vi "Func-엑셀 데이터를 그래프로 출력.vi"() -> ()   [LabVIEW 2015] (continued)
-18.3\t-18.31\t-8.468\n-18.3\t-18.31\t-8.468\n-18.3\t-18.31\t-8.468\n-18.3\t-18.31\t-8.469\n-18.3\t-18.31\t-8.468\n-18.3\t-18.31\t-8.47\n-18.3\t-18.31\t-8.471\n-18.3\t-18.31\t-8.473\n-18.3\t-18.31\t-8.477\n-18.3\t-18.31\t-8.479\n-18.3\t-18.31\t-8.48\n-18.3\t-18.31\t-8.477\n-18.3\t-18.31\t-8.477\n-18.3\t-18.31\t-8.478\n-18.3\t-18.31\t-8.474\n-18.3\t-18.31\t-8.47\n-18.3\t-18.31\t-8.47\n-18.3\t-18.31\t-8.472\n-18.3\t-18.31\t-8.475\n-18.3\t-18.31\t-8.474\n-18.3\t-18.31\t-8.478\n-18.3\t-18.31\t-8.48\n-18.3\t-18.31\t-8.48\n-18.3\t-18.31\t-8.482\n-18.3\t-18.31\t-8.481\n-18.3\t-18.31\t-8.48\n-18.3\t-18.31\t-8.48\n-18.3\t-18.31\t-8.477\n-18.3\t-18.31\t-8.48\n-18.3\t-18.31\t-8.48\n-18.3\t-18.31\t-8.483\n-18.3\t-18.31\t-8.484\n-18.3\t-18.31\t-8.484\n-18.3\t-18.31\t-8.489\n-18.3\t-18.31\t-8.49\n-18.3\t-18.31\t-8.49\n-18.3\t-18.31\t-8.489\n-18.3\t-18.31\t-8.487\n-18.3\t-18.31\t-8.486\n-18.3\t-18.31\t-8.484\n-18.3\t-18.31\t-8.481\n-18.3\t-18.31\t-8.482\n-18.3\t-18.31\t-8.484\n-18.3\t-18.31\t-8.483\n-18.3\t-18.31\t-8.486\n-18.3\t-18.31\t-8.487\n-18.3\t-18.31\t-8.489\n-18.3\t-18.31\t-8.488\n-18.3\t-18.31\t-8.484\n-18.3\t-18.31\t-8.486\n-18.3\t-18.31\t-8.487\n-18.3\t-18.31\t-8.491\n-18.3\t-18.31\t-8.491\n-18.3\t-18.31\t-8.491\n-18.3\t-18.31\t-8.495\n-18.3\t-18.31\t-8.496\n-18.3\t-18.31\t-8.492\n-18.3\t-18.31\t-8.491\n-18.3\t-18.31\t-8.493\n-18.3\t-18.31\t-8.496\n-18.3\t-18.31\t-8.495\n-18.3\t-18.31\t-8.495\n-18.3\t-18.31\t-8.496\n-18.3\t-18.31\t-8.495\n-18.3\t-18.31\t-8.497\n-18.3\t-18.31\t-8.494\n-18.3\t-18.31\t-8.495\n-18.3\t-18.31\t-8.5\n-18.3\t-18.31\t-8.499\n-18.3\t-18.31\t-8.5\n-18.3\t-18.31\t-8.499\n-18.3\t-18.31\t-8.503\n-18.3\t-18.31\t-8.507\n-18.3\t-18.31\t-8.505\n-18.3\t-18.31\t-8.507\n-18.3\t-18.31\t-8.506\n-18.3\t-18.31\t-8.506\n-18.3\t-18.31\t-8.503\n-18.3\t-18.31\t-8.502\n-18.3\t-18.31\t-8.503\n-18.3\t-18.31\t-8.503\n-18.3\t-18.31\t-8.505\n-18.3\t-18.31\t-8.504\n-18.3\t-18.31\t-8.507\n-18.3\t-18.31\t-8.502\n-18.3\t-18.31\t-8.5\n-18.3\t-18.31\t-8.502\n-18.3\t-18.31\t-8.505\n-18.3\t-18.31\t-8.508\n-18.3\t-18.31\t-8.506\n-18.3\t-18.31\t-8.508\n-18.3\t-18.31\t-8.511\n-18.3\t-18.31\t-8.514\n-18.3\t-18.31\t-8.513\n-18.3\t-18.31\t-8.512\n-18.3\t-18.31\t-8.515\n-18.3\t-18.31\t-8.517\n-18.3\t-18.31\t-8.513\n-18.3\t-18.31\t-8.509\n-18.3\t-18.31\t-8.508\n-18.3\t-18.31\t-8.509\n-18.3\t-18.31\t-8.507\n-18.3\t-18.31\t-8.507\n-18.393\t-18.38\t-8.775\n-18.477\t-18.44\t-8.782\n-18.56\t-18.33\t-8.786\n-18.643\t-18.35\t-8.786\n-18.727\t-18.4\t-8.796\n-18.81\t-18.46\t-8.785\n-18.893\t-18.53\t-8.79\n-18.977\t-18.6\t-8.793\n-19.06\t-18.68\t-8.792\n-19.143\t-18.77\t-8.794\n-19.227\t-18.87\t-8.797\n-19.31\t-18.99\t-8.789\n-19.393\t-19.09\t-8.798\n-19.477\t-19.21\t-8.807\n-19.56\t-19.33\t-8.797\n-19.643\t-19.43\t-8.805\n-19.727\t-19.53\t-8.807\n-19.81\t-19.65\t-8.809\n-19.893\t-19.77\t-8.82\n-19.977\t-19.88\t-8.813\n-20.06\t-20.01\t-8.825\n-20.143\t-20.12\t-8.83\n-20.227\t-20.24\t-8.835\n-20.31\t-20.34\t-8.841\n-20.393\t-20.46\t-8.852\n-20.477\t-20.57\t-8.857\n-20.56\t-20.68\t-8.861\n-20.643\t-20.8\t-8.873\n-20.727\t-20.9\t-8.873\n-20.81\t-21.01\t-8.89\n-20.893\t-21.11\t-8.904\n-20.977\t-21.21\t-8.911\n-21.06\t-21.33\t-8.929\n-21.143\t-21.43\t-8.927\n-21.227\t-21.54\t-8.944\n-21.31\t-21.63\t-8.961\n-21.393\t-21.71\t-8.978\n-21.477\t-21.8\t-8.993\n-21.56\t-21.87\t-9.011\n-21.643\t-21.94\t-9.028\n-21.727\t-22.01\t-9.045\n-21.81\t-22.07\t-9.071\n-21.893\t-22.14\t-9.091\n-21.977\t-22.21\t-9.109\n-22.06\t-22.28\t-9.134\n-22.143\t-22.36\t-9.152\n-22.227\t-22.45\t-9.172\n-22.31\t-22.53\t-9.2\n-22.393\t-22.6\t-9.224\n-22.477\t-22.68\t-9.25\n-22.56\t-22.76\t-9.272\n-22.643\t-22.84\t-9.297\n-22.727\t-22.92\t-9.329\n-22.81\t-22.99\t-9.355\n-22.893\t-23.07\t-9.387\n-22.977\t-23.15\t-9.423\n-23.06\t-23.22\t-9.445\n-23.143\t-23.29\t-9.477\n-23.227\t-23.36\t-9.505\n-23.31\t-23.45\t-9.534\n-23.393\t-23.53\t-9.572\n-23.477\t-23.62\t-9.603\n-23.56\t-23.69\t-9.63\n-23.643\t-23.77\t-9.668\n-23.727\t-23.85\t-9.7\n-23.81\t-23.93\t-9.739\n-23.893\t-24.01\t-9.771\n-23.977\t-24.09\t-9.805\n-24.06\t-24.17\t-9.846\n-24.143\t-24.24\t-9.882\n-24.227\t-24.31\t-9.915\n-24.31\t-24.4\t-9.965\n-24.393\t-24.49\t-10.003\n-24.477\t-24.56\t-10.039\n-24.56\t-24.64\t-10.073\n-24.643\t-24.72\t-10.12\n-24.727\t-24.81\t-10.156\n-24.81\t-24.88\t-10.202\n-24.893\t-24.96\t-10.24\n-24.977\t-25.04\t-10.284\n-25.06\t-25.1\t-10.323\n-25.143\t-25.19\t-10.372\n-25.227\t-25.27\t-10.418\n-25.31\t-25.35\t-10.457\n-25.393\t-25.42\t-10.498\n-25.477\t-25.5\t-10.549\n-25.56\t-25.58\t-10.6\n-25.643\t-25.65\t-10.641\n-25.727\t-25.74\t-10.692\n-25.81\t-25.83\t-10.733\n-25.893\t-25.91\t-10.783\n-25.977\t-26\t-10.832\n-26.06\t-26.08\t-10.873\n-26.143\t-26.15\t-10.932\n-26.227\t-26.24\t-10.976\n-26.31\t-26.32\t-11.023\n-26.393\t-26.41\t-11.073\n-26.477\t-26.48\t-11.118\n-26.56\t-26.56\t-11.17\n-26.643\t-26.65\t-11.228\n-26.727\t-26.73\t-11.275\n-26.81\t-26.81\t-11.33\n-26.893\t-26.88\t-11.382\n-26.977\t-26.96\t-11.434\n-27.06\t-27.05\t-11.488\n-27.143\t-27.13\t-11.539\n-27.227\t-27.21\t-11.586\n-27.31\t-27.29\t-11.647\n-27.393\t-27.37\t-11.699\n-27.477\t-27.45\t-11.745\n-27.56\t-27.52\t-11.804\n-27.643\t-27.62\t-11.864\n-27.727\t-27.7\t-11.916\n-27.81\t-27.79\t-11.971\n-27.893\t-27.87\t-12.027\n-27.977\t-27.95\t-12.079\n-28.06\t-28.03\t-12.136\n-28.143\t-28.11\t-12.201\n-28.227\t-28.2\t-12.257\n-28.31\t-28.27\t-12.312\n-28.393\t-28.34\t-12.365\n-28.477\t-28.41\t-12.42\n-28.56\t-28.49\t-12.481\n-28.643\t-28.57\t-12.543\n-28.727\t-28.62\t-12.597\n-28.81\t-28.69\t-12.665\n-28.893\t-28.77\t-12.714\n-28.977\t-28.84\t-12.777\n-29.06\t-28.94\t-12.842\n-29.143\t-29.01\t-12.898\n-29.227\t-29.09\t-12.951\n-29.31\t-29.16\t-13.021\n-29.393\t-29.23\t-13.081\n-29.477\t-29.3\t-13.142\n-29.56\t-29.38\t-13.202\n-29.643\t-29.47\t-13.272\n-29.727\t-29.54\t-13.326\n-29.81\t-29.61\t-13.389\n-29.893\t-29.69\t-13.455\n-29.977\t-29.75\t-13.518\n-30.06\t-29.82\t-13.585\n-30.143\t-29.89\t-13.646\n-30.227\t-29.97\t-13.701\n-30.31\t-30.04\t-13.77\n-30.393\t-30.11\t-13.834\n-30.477\t-30.17\t-13.901\n-30.56\t-30.25\t-13.957\n-30.643\t-30.33\t-14.017\n-30.727\t-30.41\t-14.083\n-30.81\t-30.47\t-14.148\n-30.893\t-30.53\t-14.214\n-30.977\t-30.61\t-14.278\n-31.06\t-30.69\t-14.342\n-31.143\t-30.77\t-14.413\n-31.227\t-30.85\t-14.474\n-31.31\t-30.93\t-14.534\n-31.393\t-30.99\t-14.599\n-31.477\t-31.07\t-14.666\n-31.56\t-31.14\t-14.736\n-31.643\t-31.2\t-14.794\n-31.727\t-31.28\t-14.858\n-31.81\t-31.34\t-14.926\n-31.893\t-31.4\t-14.989\n-31.977\t-31.47\t-15.061\n-32.06\t-31.54\t-15.121\n-32.143\t-31.59\t-15.184\n-32.227\t-31.65\t-15.247\n-32.31\t-31.72\t-15.306\n-32.393\t-31.78\t-15.383\n-32.477\t-31.84\t-15.443\n-32.56\t-31.91\t-15.514\n-32.643\t-31.98\t-15.58\n-32.727\t-32.04\t-15.645\n-32.81\t-32.12\t-15.707\n-32.893\t-32.19\t-15.763\n-32.977\t-32.26\t-15.84\n-33.06\t-32.32\t-15.909\n-33.143\t-32.38\t-15.976\n-33.227\t-32.45\t-16.038\n-33.31\t-32.5\t-16.112\n-33.393\t-32.57\t-16.169\n-33.477\t-32.63\t-16.237\n-33.56\t-32.71\t-16.298\n-33.643\t-32.77\t-16.368\n-33.727\t-32.83\t-16.44\n-33.81\t-32.89\t-16.507\n-33.893\t-32.95\t-16.564\n-33.977\t-33.01\t-16.636\n-34.06\t-33.07\t-16.703\n-34.143\t-33.13\t-16.773\n-34.227\t-33.18\t-16.849\n-34.31\t-33.24\t-16.907\n-34.393\t-33.3\t-16.971\n-34.477\t-33.35\t-17.047\n-34.56\t-33.42\t-17.107\n-34.643\t-33.48\t-17.175\n-34.727\t-33.55\t-17.237\n-34.81\t-33.6\t-17.304\n-34.893\t-33.65\t-17.37\n-34.977\t-33.71\t-17.43\n-35.06\t-33.77\t-17.502\n-35.143\t-33.81\t-17.574\n-35.227\t-33.87\t-17.633\n-35.31\t-33.93\t-17.701\n-35.393\t-33.99\t-17.767\n-35.477\t-34.04\t-17.843\n-35.56\t-34.1\t-17.901\n-35.643\t-34.17\t-17.968\n-35.727\t-34.23\t-18.035\n-35.81\t-34.28\t-18.101\n-35.893\t-34.33\t-18.162\n-35.977\t-34.39\t-18.234\n-36.06\t-34.45\t-18.304\n-36.143\t-34.51\t-18.366\n-36.227\t-34.57\t-18.426\n-36.31\t-34.62\t-18.493\n-36.393\t-34.69\t-18.558\n-36.477\t-34.74\t-18.622\n-36.56\t-34.79\t-18.701\n-36.643\t-34.84\t-18.761\n-36.727\t-34.9\t-18.83\n-36.81\t-34.96\t-18.904\n-36.893\t-35.02\t-18.953\n-36.977\t-35.07\t-19.021\n-37.06\t-35.12\t-19.084\n-37.143\t-35.17\t-19.152\n-37.227\t-35.22\t-19.221\n-37.31\t-35.28\t-19.285\n-37.393\t-35.33\t-19.348\n-37.477\t-35.38\t-19.409\n-37.56\t-35.44\t-19.473\n-37.643\t-35.5\t-19.538\n-37.727\t-35.56\t-19.6\n-37.81\t-35.61\t-19.672\n-37.893\t-35.67\t-19.735\n-37.977\t-35.73\t-19.793\n-38.06\t-35.77\t-19.856\n-38.143\t-35.83\t-19.925\n-38.227\t-35.87\t-19.992\n-38.31\t-35.91\t-20.059\n-38.393\t-35.97\t-20.12\n-38.477\t-36.03\t-20.18\n-38.56\t-36.08\t-20.245\n-38.643\t-36.13\t-20.312\n-38.727\t-36.18\t-20.375\n-38.81\t-36.22\t-20.427\n-38.893\t-36.29\t-20.506\n-38.977\t-36.33\t-20.566\n-39.06\t-36.38\t-20.625\n-39.143\t-36.44\t-20.691\n-39.227\t-36.5\t-20.754\n-39.31\t-36.55\t-20.818\n-39.393\t-36.6\t-20.882\n-39.477\t-36.65\t-20.931\n-39.56\t-36.71\t-21.005\n-39.643\t-36.77\t-21.066\n-39.727\t-36.82\t-21.126\n-39.81\t-36.88\t-21.179\n-39.893\t-36.93\t-21.246\n-39.977\t-36.98\t-21.304\n-40.06\t-37.04\t-21.37\n-40\t-37.1\t-21.425\n-40\t-37.1\t-21.426\n-40\t-37.11\t-21.432\n-40\t-37.11\t-21.436\n-40\t-37.11\t-21.443\n-40\t-37.12\t-21.441\n-40\t-37.13\t-21.448\n-40\t-37.13\t-21.453\n-40\t-37.14\t-21.456\n-40\t-37.15\t-21.467\n-40\t-37.16\t-21.473\n-40\t-37.16\t-21.486\n-40\t-37.17\t-21.496\n-40\t-37.17\t-21.499\n-40\t-37.17\t-21.505\n-40\t-37.18\t-21.511\n-40\t-37.18\t-21.516\n-40\t-37.18\t-21.52\n-40\t-37.18\t-21.521\n-40\t-37.19\t-21.527\n-40\t-37.19\t-21.534\n-40\t-37.19\t-21.543\n-40\t-37.2\t-21.549\n-40\t-37.2\t-21.555\n-40\t-37.2\t-21.564\n-40\t-37.21\t-21.571\n-40\t-37.21\t-21.573\n-40\t-37.22\t-21.578\n-40\t-37.22\t-21.583\n-40\t-37.23\t-21.59\n-40\t-37.23\t-21.598\n-40\t-37.24\t-21.605\n-40\t-37.24\t-21.613\n-40\t-37.25\t-21.616\n-40\t-37.25\t-21.618\n-40\t-37.25\t-21.623\n-40\t-37.26\t-21.628\n-40\t-37.26\t-21.631\n-40\t-37.26\t-21.638\n-40\t-37.26\t-21.648\n-40\t-37.27\t-21.655\n-40\t-37.27\t-21.664\n-40\t-37.28\t-21.672\n-40\t-37.28\t-21.679\n-40\t-37.29\t-21.686\n-40\t-37.3\t-21.687\n-40\t-37.3\t-21.695\n-40\t-37.31\t-21.696\n-40\t-37.32\t-21.7\n-40\t-37.32\t-21.707\n-40\t-37.33\t-21.715\n-40\t-37.33\t-21.725\n-40\t-37.33\t-21.73\n-40\t-37.33\t-21.741\n-40\t-37.34\t-21.746\n-40\t-37.34\t-21.753\n-40\t-37.35\t-21.759\n-40\t-37.36\t-21.764\n-40\t-37.36\t-21.772\n-40\t-37.37\t-21.777\n-40\t-37.37\t-21.781\n-40\t-37.38\t-21.785\n-40\t-37.38\t-21.795\n-40\t-37.39\t-21.802\n-40\t-37.4\t-21.805\n-40\t-37.4\t-21.816\n-40\t-37.41\t-21.821\n-40\t-37.41\t-21.824\n-40\t-37.41\t-21.829\n-40\t-37.41\t-21.831\n-40\t-37.42\t-21.837\n-40\t-37.42\t-21.843\n-40\t-37.43\t-21.849\n-40\t-37.43\t-21.859\n-40\t-37.44\t-21.869\n-40\t-37.44\t-21.879\n-40\t-37.45\t-21.883\n-40\t-37.45\t-21.892\n-40\t-37.46\t-21.896\n-40\t-37.47\t-21.898\n-40\t-37.47\t-21.902\n-40\t-37.48\t-21.901\n-40\t-37.48\t-21.904\n-40\t-37.48\t-21.909\n-40\t-37.49\t-21.916\n-40\t-37.49\t-21.921\n-40\t-37.49\t-21.927\n-40\t-37.49\t-21.937\n-40\t-37.5\t-21.947\n-40\t-37.51\t-21.956\n-40\t-37.52\t-21.961\n-40\t-37.53\t-21.966\n-40\t-37.54\t-21.977\n-40\t-37.54\t-21.978\n-40\t-37.55\t-21.98\n-40\t-37.56\t-21.986\n-40\t-37.56\t-21.989\n-40\t-37.57\t-21.995\n-40\t-37.57\t-22.001\n-40\t-37.58\t-22.008\n-40\t-37.59\t-22.015\n-40\t-37.59\t-22.022\n-40\t-37.6\t-22.027\n-40\t-37.61\t-22.035\n-40\t-37.61\t-22.039\n-40\t-37.62\t-22.048\n-40\t-37.63\t-22.052\n-40\t-37.63\t-22.061\n-40\t-37.63\t-22.066\n-40\t-37.64\t-22.071\n-40\t-37.64\t-22.076\n-40\t-37.64\t-22.079\n-40\t-37.64\t-22.086\n-40\t-37.65\t-22.088\n-40\t-37.65\t-22.096\n-40\t-37.66\t-22.105\n-40\t-37.66\t-22.111\n-40\t-37.67\t-22.118\n-40\t-37.67\t-22.125\n-40\t-37.68\t-22.132\n-40\t-37.68\t-22.138\n-40\t-37.69\t-22.145\n-40\t-37.69\t-22.154\n-40\t-37.7\t-22.157\n-40\t-37.71\t-22.165\n-40\t-37.71\t-22.168\n-40\t-37.71\t-22.17\n-40\t-37.71\t-22.177\n-40\t-37.71\t-22.18\n-40\t-37.72\t-22.186\n-40\t-37.72\t-22.192\n-40\t-37.73\t-22.198\n-40\t-37.74\t-22.203\n-40\t-37.75\t-22.207\n-40\t-37.75\t-22.213\n-40\t-37.76\t-22.219\n-40\t-37.77\t-22.227\n-40\t-37.77\t-22.233\n-40\t-37.78\t-22.241\n-40\t-37.78\t-22.251\n-40\t-37.79\t-22.256\n-40\t-37.79\t-22.263\n-40\t-37.79\t-22.271\n-40\t-37.79\t-22.276\n-40\t-37.8\t-22.279\n-40\t-37.8\t-22.286\n-40\t-37.81\t-22.289\n-40\t-37.82\t-22.294\n-40\t-37.82\t-22.298\n-40\t-37.83\t-22.306\n-40\t-37.83\t-22.31\n-40\t-37.84\t-22.318\n-40\t-37.84\t-22.325\n-40\t-37.85\t-22.33\n-40\t-37.86\t-22.341\n-40\t-37.86\t-22.342\n-40\t-37.86\t-22.346\n-40\t-37.87\t-22.352\n-40\t-37.87\t-22.358\n-40\t-37.88\t-22.362\n-40\t-37.88\t-22.369\n-40\t-37.88\t-22.377\n-40\t-37.89\t-22.386\n-40\t-37.9\t-22.393\n-40\t-37.91\t-22.398\n-40\t-37.91\t-22.403\n-40\t-37.92\t-22.408\n-40\t-37.92\t-22.413\n-40\t-37.93\t-22.42\n-40\t-37.93\t-22.43\n-40\t-37.93\t-22.432\n-40\t-37.94\t-22.441\n-40\t-37.94\t-22.447\n-40\t-37.94\t-22.453\n-40\t-37.95\t-22.454\n-40\t-37.95\t-22.458\n-40\t-37.96\t-22.466\n-40\t-37.97\t-22.47\n-40\t-37.97\t-22.476\n-40\t-37.98\t-22.482\n-40\t-37.98\t-22.492\n-40\t-37.99\t-22.496\n-40\t-37.99\t-22.5\n-40\t-38\t-22.505\n-40\t-38.01\t-22.511\n-40\t-38.01\t-22.515\n-40\t-38.01\t-22.521\n-40\t-38.02\t-22.527\n-40\t-38.03\t-22.533\n-40\t-38.03\t-22.541\n-40\t-38.04\t-22.548\n-40\t-38.05\t-22.553\n-40\t-38.05\t-22.558\n-40\t-38.06\t-22.566\n-40\t-38.07\t-22.57\n-40\t-38.08\t-22.574\n-40\t-38.08\t-22.583\n-40\t-38.08\t-22.59\n-40\t-38.09\t-22.6\n-40\t-38.1\t-22.607\n-40\t-38.11\t-22.611\n-40\t-38.12\t-22.618\n-40\t-38.12\t-22.622\n-40\t-38.13\t-22.625\n-40\t-38.14\t-22.632\n-40\t-38.14\t-22.636\n-40\t-38.15\t-22.642\n-40\t-38.16\t-22.648\n-40\t-38.16\t-22.655\n-40\t-38.16\t-22.659\n-40\t-38.16\t-22.664\n-40\t-38.17\t-22.665\n-40\t-38.17\t-22.675\n-40\t-38.18\t-22.682\n-40\t-38.18\t-22.687\n-40\t-38.18\t-22.692\n-40\t-38.19\t-22.704\n-40\t-38.19\t-22.712\n-40\t-38.19\t-22.715\n-40\t-38.2\t-22.723\n-40\t-38.2\t-22.726\n-40\t-38.21\t-22.733\n-40\t-38.22\t-22.735\n-40\t-38.22\t-22.739\n-40\t-38.23\t-22.745\n-40\t-38.23\t-22.752\n-40\t-38.24\t-22.755\n-40\t-38.24\t-22.759\n-40\t-38.24\t-22.765\n-40\t-38.24\t-22.773\n-40\t-38.24\t-22.779\n-40\t-38.25\t-22.786\n-40\t-38.25\t-22.793\n-40\t-38.26\t-22.8\n-40\t-38.27\t-22.809\n-40\t-38.27\t-22.812\n-40\t-38.28\t-22.817\n-40\t-38.28\t-22.825\n-40\t-38.29\t-22.834\n-40\t-38.29\t-22.835\n-40\t-38.3\t-22.845\n-40\t-38.3\t-22.848\n-40\t-38.31\t-22.85\n-40\t-38.31\t-22.857\n-40\t-38.31\t-22.859\n-40\t-38.31\t-22.865\n-40\t-38.31\t-22.871\n-40\t-38.32\t-22.878\n-40\t-38.33\t-22.887\n-40\t-38.33\t-22.891\n-40\t-38.34\t-22.896\n-40\t-38.34\t-22.902\n-40\t-38.34\t-22.906\n-40\t-38.35\t-22.91\n-40\t-38.35\t-22.914\n-40\t-38.35\t-22.925\n-40\t-38.36\t-22.93\n-40\t-38.36\t-22.938\n-40\t-38.36\t-22.948\n-40\t-38.37\t-22.956\n-40\t-38.37\t-22.96\n-40\t-38.37\t-22.968\n-40\t-38.38\t-22.973\n-40\t-38.38\t-22.978\n-40\t-38.38\t-22.984\n-40\t-38.39\t-22.987\n-40\t-38.39\t-22.995\n-40\t-38.4\t-23\n-40\t-38.4\t-23.009\n-40\t-38.41\t-23.013\n-40\t-38.41\t-23.018\n-40\t-38.42\t-23.024\n-40\t-38.42\t-23.031\n-40\t-38.43\t-23.037\n-40\t-38.43\t-23.041\n-40\t-38.44\t-23.048\n-40\t-38.44\t-23.054\n-40\t-38.44\t-23.061\n-40\t-38.45\t-23.066\n-40\t-38.45\t-23.072\n-40\t-38.46\t-23.074\n-40\t-38.46\t-23.08\n-40\t-38.46\t-23.082\n-40\t-38.47\t-23.085\n-40\t-38.47\t-23.088\n-40\t-38.48\t-23.093\n-40\t-38.49\t-23.101\n-40\t-38.5\t-23.11\n-40\t-38.5\t-23.117\n-40\t-38.51\t-23.123\n-40\t-38.52\t-23.13\n-40\t-38.53\t-23.134\n-40\t-38.53\t-23.138\n-40\t-38.54\t-23.143\n-40\t-38.54\t-23.145\n-40\t-38.55\t-23.149\n-40\t-38.55\t-23.157\n-40\t-38.56\t-23.167\n-40\t-38.56\t-23.175\n-40\t-38.57\t-23.184\n-40\t-38.57\t-23.19\n-40\t-38.58\t-23.197\n-40\t-38.59\t-23.201\n-40\t-38.6\t-23.203\n-40\t-38.61\t-23.205\n-40\t-38.61\t-23.21\n-40\t-38.61\t-23.217\n-40\t-38.62\t-23.219\n-40\t-38.62\t-23.227\n-40\t-38.63\t-23.231\n-40\t-38.63\t-23.237\n-40\t-38.64\t-23.245\n-40\t-38.65\t-23.252\n-40\t-38.65\t-23.26\n-40\t-38.66\t-23.27\n-40\t-38.66\t-23.279\n-40\t-38.67\t-23.283\n-40\t-38.67\t-23.29\n-40\t-38.68\t-23.293\n-40\t-38.68\t-23.298\n-40\t-38.68\t-23.302\n-40\t-38.68\t-23.307\n-40\t-38.69\t-23.314\n-40\t-38.69\t-23.321\n-40\t-38.7\t-23.327\n-40\t-38.7\t-23.334\n-40\t-38.71\t-23.342\n-40\t-38.72\t-23.346\n-40\t-38.72\t-23.35\n-40\t-38.73\t-23.355\n-40\t-38.74\t-23.359\n-40\t-38.74\t-23.364\n-40\t-38.75\t-23.369\n-40\t-38.75\t-23.373\n-40\t-38.75\t-23.379\n-40\t-38.75\t-23.385\n-40\t-38.76\t-23.389\n-40\t-38.76\t-23.394\n-40\t-38.77\t-23.403\n-40\t-38.77\t-23.407\n-40\t-38.78\t-23.411\n-40\t-38.78\t-23.42\n-40\t-38.79\t-23.423\n-40\t-38.8\t-23.43\n-40\t-38.8\t-23.436\n-40\t-38.81\t-23.443\n-40\t-38.82\t-23.45\n-40\t-38.82\t-23.456\n-40\t-38.83\t-23.462\n-40\t-38.83\t-23.468\n-40\t-38.83\t-23.474\n-40\t-38.83\t-23.479\n-40\t-38.84\t-23.481\n-40\t-38.85\t-23.491\n-40\t-38.85\t-23.495\n-40\t-38.86\t-23.5\n-40\t-38.87\t-23.509\n-40\t-38.87\t-23.513\n-40\t-38.88\t-23.519\n-40\t-38.88\t-23.525\n-40\t-38.89\t-23.53\n-40\t-38.89\t-23.535\n-40\t-38.9\t-23.542\n-40\t-38.9\t-23.547\n-40\t-38.9\t-23.554\n-40\t-38.91\t-23.561\n-40\t-38.91\t-23.569\n-40\t-38.92\t-23.572\n-40\t-38.92\t-23.577\n-40\t-38.93\t-23.584\n-40\t-38.93\t-23.586\n-40\t-38.93\t-23.589\n-40\t-38.94\t-23.593\n-40\t-38.94\t-23.597\n-40\t-38.95\t-23.608\n-40\t-38.95\t-23.61\n-40\t-38.96\t-23.616\n-40\t-38.96\t-23.626\n-40\t-38.97\t-23.632\n-40\t-38.97\t-23.636\n-40\t-38.98\t-23.641\n-40\t-38.98\t-23.647\n-40\t-38.99\t-23.654\n-40\t-38.99\t-23.657\n-40\t-38.99\t-23.662\n-40\t-39\t-23.667\n-40\t-39\t-23.671\n-40\t-39.01\t-23.678\n-40\t-39.01\t-23.682\n-40\t-39.02\t-23.689\n-40\t-39.02\t-23.695\n-40\t-39.03\t-23.704\n-40\t-39.03\t-23.713\n-40\t-39.04\t-23.713\n-40\t-39.05\t-23.72\n-40\t-39.05\t-23.732\n-40\t-39.06\t-23.734\n-40\t-39.06\t-23.735\n-40\t-39.06\t-23.741\n-40\t-39.06\t-23.749\n-40\t-39.07\t-23.753\n-40\t-39.07\t-23.757\n-40\t-39.08\t-23.764\n-40\t-39.09\t-23.771\n-40\t-39.09\t-23.779\n-40\t-39.1\t-23.786\n-40\t-39.1\t-23.791\n-40\t-39.1\t-23.799\n-40\t-39.11\t-23.804\n-40\t-39.11\t-23.812\n-40\t-39.12\t-23.816\n-40\t-39.12\t-23.821\n-40\t-39.13\t-23.828\n-40\t-39.13\t-23.83\n-40\t-39.13\t-23.836\n-40\t-39.13\t-23.836\n-40\t-39.14\t-23.842\n-40\t-39.14\t-23.844\n-40\t-39.15\t-23.848\n-40\t-39.16\t-23.857\n-40\t-39.16\t-23.862\n-40\t-39.17\t-23.869\n-40\t-39.17\t-23.878\n-40\t-39.18\t-23.886\n-40\t-39.18\t-23.894\n-40\t-39.19\t-23.902\n-40\t-39.19\t-23.904\n-40\t-39.2\t-23.911\n-40\t-39.2\t-23.915\n-40\t-39.2\t-23.918\n-40\t-39.21\t-23.924\n-40\t-39.21\t-23.932\n-40\t-39.22\t-23.94\n-40\t-39.23\t-23.943\n-40\t-39.24\t-23.95\n-40\t-39.24\t-23.959\n-40\t-39.25\t-23.96\n-40\t-39.25\t-23.966\n-40\t-39.26\t-23.97\n-40\t-39.26\t-23.979\n-40\t-39.27\t-23.986\n-40\t-39.28\t-23.986\n-40\t-39.28\t-23.993\n-40\t-39.29\t-24.001\n-40\t-39.29\t-24.004\n-40\t-39.29\t-24.006\n-40\t-39.29\t-24.013\n-40\t-39.29\t-24.019\n-40\t-39.3\t-24.024\n-40\t-39.3\t-24.029\n-40\t-39.31\t-24.037\n-40\t-39.32\t-24.045\n-40\t-39.32\t-24.05\n-40\t-39.32\t-24.054\n-40\t-39.33\t-24.057\n-40\t-39.33\t-24.065\n-40\t-39.34\t-24.071\n-40\t-39.34\t-24.073\n-40\t-39.35\t-24.08\n-40\t-39.35\t-24.091\n-40\t-39.35\t-24.097\n-40\t-39.35\t-24.102\n-40\t-39.35\t-24.105\n-40\t-39.36\t-24.111\n-40\t-39.36\t-24.116\n-40\t-39.37\t-24.119\n-40\t-39.37\t-24.123\n-40\t-39.38\t-24.13\n-40\t-39.38\t-24.136\n-40\t-39.38\t-24.14\n-40\t-39.39\t-24.151\n-40\t-39.39\t-24.156\n-40\t-39.4\t-24.161\n-40\t-39.4\t-24.17\n-40\t-39.4\t-24.175\n-40\t-39.41\t-24.182\n-40\t-39.41\t-24.185\n-40\t-39.41\t-24.191\n-40\t-39.42\t-24.2\n-40\t-39.42\t-24.205\n-40\t-39.42\t-24.21\n-40\t-39.43\t-24.214\n-40\t-39.43\t-24.223\n-40\t-39.43\t-24.229\n-40\t-39.43\t-24.231\n-40\t-39.44\t-24.237\n-40\t-39.44\t-24.24\n-40\t-39.44\t-24.245\n-40\t-39.45\t-24.252\n-40\t-39.45\t-24.254\n-40\t-39.45\t-24.259\n-40\t-39.46\t-24.267\n-40\t-39.46\t-24.275\n-40\t-39.46\t-24.28\n-40\t-39.47\t-24.286\n-40\t-39.47\t-24.292\n-40\t-39.47\t-24.296\n-40\t-39.48\t-24.302\n-40\t-39.48\t-24.306\n-40\t-39.48\t-24.309\n-40\t-39.48\t-24.315\n-40\t-39.49\t-24.32\n-40\t-39.49\t-24.326\n-40\t-39.5\t-24.334\n-40\t-39.5\t-24.34\n-40\t-39.5\t-24.348\n-40\t-39.5\t-24.355\n-40\t-39.5\t-24.361\n-40\t-39.5\t-24.367\n
